vi "ReadPLC_Keyence.vi"(9 "MemoryNumber":string, 11 "IP Address":string) -> (1 "BoolRead":bool)   [LabVIEW 2017]
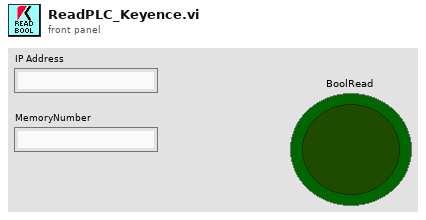
[diagram p1: front panel]
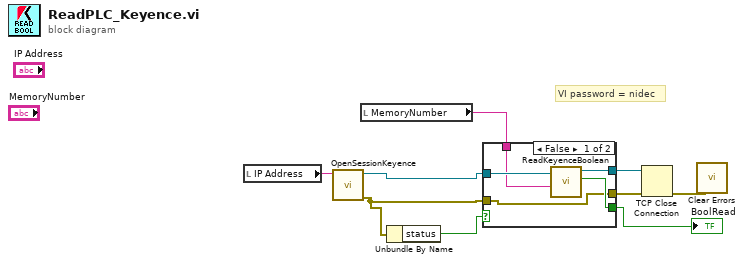
[diagram p0: block diagram]
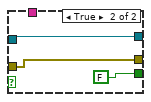
[diagram p2: hidden frame]
diagram:
  # "VI password = nidec"
  n1 = local read "IP Address"() -> (w8:string)
  n2 = call "OpenSessionKeyence.vi"("address"=w8) -> ("error out"=w4:errorcluster, "TCP Network Connection out"=w7:refnum<k5>)  [unwired: 9 in]
  n3 = local read "MemoryNumber"() -> (w1:string)
  n4 = Unbundle By Name(w4) -> ("status"=w5:bool)
  n5 = case shown="False" w5 {
    tunnel: [w14 FALSE] -> w9
    tunnel: w7 -> [w13 w17]
    tunnel: [w12 w17] -> w6
    tunnel: w4 -> [w11 w16]
    tunnel: [w11 w16] -> w3
    tunnel: w1 -> [w10 _]
    frame False {
      n6 = call "ReadKeyenceBoolean.vi"("MemoryNumber"=w10, "connection ID"=w13) -> ("status"=w14:bool, "connection ID out"=w12:refnum<k5>)  [unwired: 8 in]
    }
    frame True {
    }
  }
  "BoolRead" <- w9
  n7 = TCP Close Connection(connection ID=w6, error in (no error)=w3) -> (error out=w2:errorcluster)  [unwired: 1 in, 1 out]
  n8 = call <vilib>:"Clear Errors.vi"("error in (no error)"=w2) -> ()  [unwired: 5 in, 2 out]
